vi "4-4.vi"(0 "duration (msec)":u32 caption="持续时间（毫秒）", 1 "数值":dbl, 2 "use system alert? (T)":bool=TRUE caption="使用系统警报？(T)", 3 "frequency (Hz)":u32 caption="频率(Hz)") -> ()   [LabVIEW 2017]
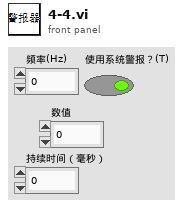
[diagram p1: front panel]
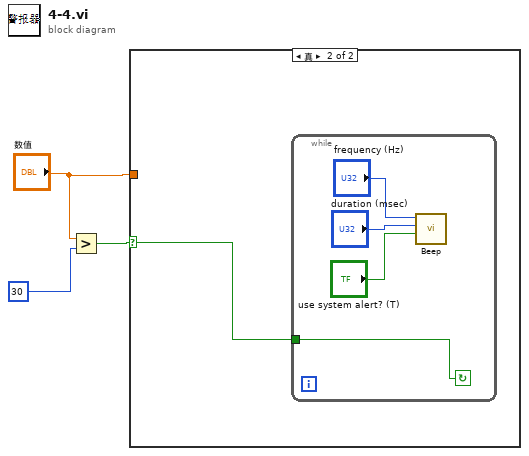
[diagram p0: block diagram]
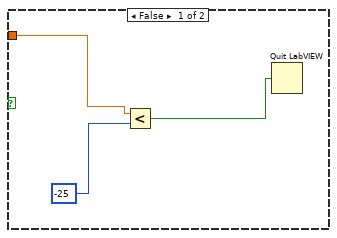
[diagram p2: hidden frame]
diagram:
  n1 = Greater?(x="数值", y=30) -> (0:w2:bool)
  n2 = case shown="真" w2 {
    selector: w2 -> [_ w7]
    tunnel: "数值" -> [w4 _]
    frame False {
      n3 = Less?(x=w4, y=-25) -> (x < y?=w5:bool)
      n4 = Quit LabVIEW(quit? (T)=w5) -> ()
    }
    frame True {
      n5 = while {
        tunnel: w7 -> [w8]
        stop <- w8 continue-if-true
        n6 = call <vilib>:"Beep.vi"("use system alert? (T)"="use system alert? (T)", "duration (msec)"="duration (msec)", "frequency (Hz)"="frequency (Hz)") -> ()  [unwired: 9 in]
      }
    }
  }
